vi "Send Pre-Addressed Publish.vi"(8 "error in (no error)":errorcluster, 10 "PublishRequest":refnum<class "PublishRequest.lvclass">, 11 "Publish Message":refnum<class "Publish Msg.lvclass">) -> (0 "error out":errorcluster)   [LabVIEW 2019, in "IMediator.lvlib" / "Publish Msg.lvclass"]
doc: "Most Actors or VIs that want to publish data will do so with this send VI. Actors who call this method must have been given a pre-addressed Publish Msg prior to the act of sending. (For Actors, this means that they were launched with a pre-addressed Publish Msg or sent one after the Mediator came alive.)\n\n<License>\nCopyright © 2017 Composed Systems, LLC | All rights reserved\nwww.composed.io\n\nAuthor: Ethan Stern <ethan.stern@composed.io>\n\nThis software is provided \"AS IS\" WITHOUT WARRANTIES, either express or implied, AND IS FOR EDUCATIONAL PURPOSES ONLY.\n</License>"
uses:
  <vilib>/gpm_packages/@cs/mva-core/Source/IMediator/IMediator Messages/Publish Msg/Publish Msg.lvclass
  C:/Program Files/National Instruments/LabVIEW 2019/vi.lib/gpm_packages/@cs/actor-framework-messages/Source/RoundTripMessage/RoundTripMessage.lvclass
  <vilib>/gpm_packages/@cs/mva-core/Source/IMediator/PublishRequest/PublishRequest.lvclass
  <vilib>/gpm_packages/@cs/mva-core/Source/IMediator/IMediator Messages/Publish Msg/Publish Msg.lvclass/Publish Msg.ctl
  <vilib>/gpm_packages/@cs/actor-framework-messages/Source/RoundTripMessage/RoundTripMessage.lvclass/RoundTripMessage.ctl
  <vilib>/ActorFramework/Message Enqueuer/Message Enqueuer.lvclass/Message Enqueuer.ctl
  <vilib>/ActorFramework/Message Enqueuer/Enqueue.vi
  <vilib>/gpm_packages/@cs/actor-framework-messages/Source/RoundTripMessage/RoundTripMessage.lvclass
  C:/Program Files/National Instruments/LabVIEW 2019/vi.lib/ActorFramework/Message/Message.lvclass
  <vilib>/ActorFramework/Message Priority Queue/Priority Enqueue.vi
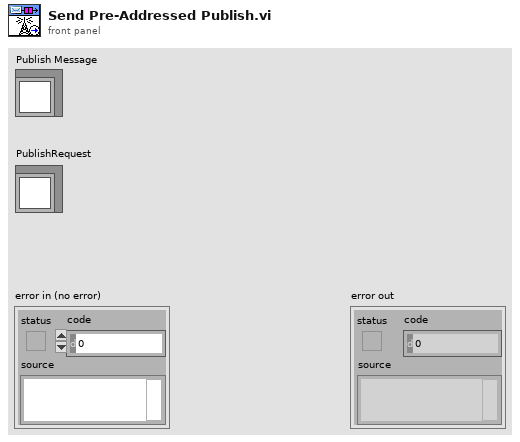
[diagram p1: front panel]
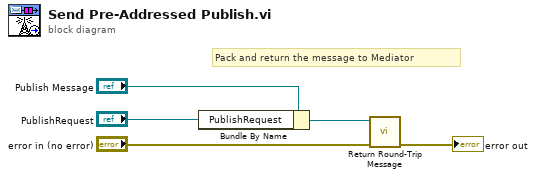
[diagram p0: block diagram]
diagram:
  # "Pack and return the message to Mediator"
  n1 = Bundle By Name(cluster="Publish Message", "PublishRequest"="PublishRequest") -> (w4:refnum<class "Publish Msg.lvclass">)
  n2 = call <vilib>:"Return Round-Trip Message.vi"("error in (no error)"="error in (no error)", "RoundTripMessage In"=w4) -> ("error out"=→"error out":errorcluster)  [unwired: 9 in]
